vi "Read SCH Parameters MGI RWA.vi"(8 "error in (no error)":errorcluster, 10 "Done":bool, 11 "FPGA Refnum in":T2) -> (0 "error out":errorcluster, 3 "Refnum out":T2)   [LabVIEW 2018]
doc: "Author: Scott Hannahs <sth@magnet.fsu.edu>\nCopyright 2018 Florida State University, All rights reserved."
uses:
  RT Controls/FPGA SCH Digitizer Ref.ctl
  SCH Data Controls/FPGA Configure Parameters.ctl
  <userlib>/_MGI/Read Write Anything/MGI RWA Options Cluster.ctl
panel:
  in  "FPGA Configuration Values":T1={"Ln2 Filter Size"=10, "VT Quench Tick Limit"=4000000, "VT Quench Volt Limit"=0.1000061035156, "Joint Tick Limit"=4000000, "Joint Volt Limit"=0.003, "CoWound Volt Limit"=0.2000122070312, "CoWound Tick Limit"=4000000, "SC Bus Limit"=0.0004000067710876, "SC Bus Tick Limit"=4000000, "ResMag Tick Limit"=1000000, "DAQ Cycle Ticks"=4096, "Res Mag dI/dt Delay"=256, "dI/dT scaling"=38.14697265625, "Pressure Inlet Limit (BarA)"=6.0, "Bore Tube Volt Limit"=0.5999999940395, "Pressure Outlet Limit (BarA)"=5.0, "Activation Current (kA)"=0.5, "Dump Resistor Scale Factor"=250.0625, "Co-Wound Asymmetry Factor"=-0.0026654, "Co-Wound Scale Factor"=60.04379999638, "Layer Scale Factors"=[4.000479996204, 3.501155003905, 3.50127799809, 3.501155003905, 3.001561000943, 3.001561000943, 3.50005300343, 3.500664994121, 3.501155003905, 4.000159993768, 3.999679997563, 4.000159993768, 3.998879998922, 3.999520003796, 3.999679997563, 4.000320002437, 4.00096000731, 4.000640004873], "Fudge Factors"=[0.0486624, 0.0491151, -0.0418637, -0.0149169, 0.0726134, -0.0451977, -0.0032112, -0.0234927, -0.002501, 0.0285479, -0.0270486, 0.003522, 0.0059306, -0.0088003, -0.0297659, 0.0390219], "Joint Scale Factors"=[0.0002005249261856, 0.0002005249261856, 0.0002004057168961, 0.000200480222702, 0.0002004057168961, 0.0002007633447647, 0.0002006888389587, 0.0002006441354752], "SC Bus Scale"=[0.100018, 0.100015, 0.00099996, 0.00099996, 0.0002005249261856, 0.0002006441354752], "Pressure Scale Factor"=[1.723690003157, 1.723690003157, 1.723690003157, 1.723690003157], "# Consecutive Zeros Fault"=1000, "Digitize Convert Ticks"=200, "Digitize Reset Ticks"=400, "Convert Clock Ticks"=20, "Digitize Read Delay Ticks"=38, "Digitize # Bits"=16, "HTS Lead Tick Limit"=4000000, "Res Lead Tick Limit"=4000000, "HTS Lead Trip"=0.1500000059605, "Res Lead Limit"=0.001953125, "HTS Lead FRZ"=0.006999999284744, "HTS Lead Warn"=0.001000002026558, "Low Current (kA)"=0.04500000178814, "Low Current Ticks"=400000000, "Low Current Delay Factor"=100, "HTS Resistance (nOhm)"=[118.0, 131.0], "Ticks to Close Relief"=80000000, "All Breaker Tick Limit"=400000000, "HTS Offset (microV)"=[0.0, 0.0], "Delay Ticks Between Bkr Reset"=1200000000, "Breaker Reset Ticks"=400000000, "PS Enable Reset Ticks"=400000000, "Reset Digitizer Ticks"=400000000, "Pressure Inlet Cooldown Limit"=12.0, "Pressure Outlet Cooldown Limit"=10.0, "Notification Email"="sth@magnet.fsu.edu"} {"Pressure Outlet Cooldown Limit" format="%.5g"; "Pressure Inlet Cooldown Limit" format="%.5g"; "HTS Offset (microV)" format="%_6g"; "HTS Resistance (nOhm)" format="%_6g"; "HTS Lead Warn" format="%_6g"; "HTS Lead FRZ" format="%_6g"; "Res Lead Limit" format="%_6g"; "HTS Lead Trip" format="%_6g"; "Pressure Scale Factor" format="%_6g"; "Joint Scale Factors" format="%_6g"; "Fudge Factors" format="%.7g"; "Co-Wound Asymmetry Factor" format="%.8g"; "Activation Current (kA)" format="%_6g"; "Pressure Outlet Limit (BarA)" format="%.5g"; "Bore Tube Volt Limit" format="%_6g"; "Pressure Inlet Limit (BarA)" format="%.5g"; "dI/dT scaling" format="%.11g"; "SC Bus Limit" format="%_6g"; "Joint Volt Limit" format="%_6g"; "VT Quench Volt Limit" format="%.5g"}
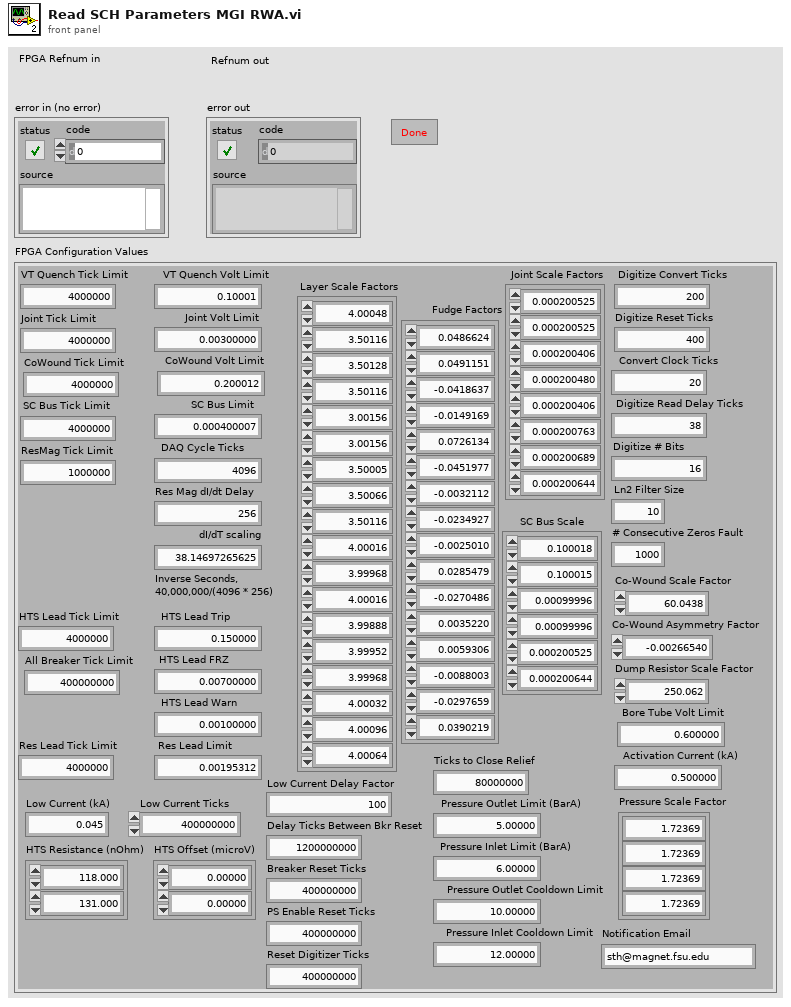
[diagram p1: front panel]
types:
  T1 = typedef "FPGA Configure Parameters.ctl" = cluster{"Ln2 Filter Size":i16, "VT Quench Tick Limit":u32, "VT Quench Volt Limit":dbl, "Joint Tick Limit":u32, "Joint Volt Limit":dbl, "CoWound Volt Limit":dbl, "CoWound Tick Limit":u32, "SC Bus Limit":dbl, "SC Bus Tick Limit":u32, "ResMag Tick Limit":u32, "DAQ Cycle Ticks":u32, "Res Mag dI/dt Delay":u32, "dI/dT scaling":dbl, "Pressure Inlet Limit (BarA)":dbl, "Bore Tube Volt Limit":dbl, "Pressure Outlet Limit (BarA)":dbl, "Activation Current (kA)":dbl, "Dump Resistor Scale Factor":dbl, "Co-Wound Asymmetry Factor":dbl, "Co-Wound Scale Factor":dbl, "Layer Scale Factors":dbl[], "Fudge Factors":dbl[], "Joint Scale Factors":dbl[], "SC Bus Scale":dbl[], "Pressure Scale Factor":dbl[], "# Consecutive Zeros Fault":i16, "Digitize Convert Ticks":u32, "Digitize Reset Ticks":u32, "Convert Clock Ticks":u32, "Digitize Read Delay Ticks":u32, "Digitize # Bits":u32, "HTS Lead Tick Limit":u32, "Res Lead Tick Limit":u32, "HTS Lead Trip":dbl, "Res Lead Limit":dbl, "HTS Lead FRZ":dbl, "HTS Lead Warn":dbl, "Low Current (kA)":dbl, "Low Current Ticks":u32, "Low Current Delay Factor":u16, "HTS Resistance (nOhm)":dbl[], "Ticks to Close Relief":u32, "All Breaker Tick Limit":u32, "HTS Offset (microV)":dbl[], "Delay Ticks Between Bkr Reset":u32, "Breaker Reset Ticks":u32, "PS Enable Reset Ticks":u32, "Reset Digitizer Ticks":u32, "Pressure Inlet Cooldown Limit":dbl, "Pressure Outlet Cooldown Limit":dbl, "Notification Email":string}
  T2 = typedef "FPGA SCH Digitizer Ref.ctl" = refnum<k20>
  T3 = typedef "MGI RWA Options Cluster.ctl" = cluster{"TS Fmt":string, "Int Fmt":string, "Delimiter":string}
  T4 = cluster{"Ln2 Filter Size":i16, "VT Quench Tick Limit":u32, "VT Quench Volt Limit":dbl, "Joint Tick Limit":u32, "Joint Volt Limit":dbl, "CoWound Volt Limit":dbl, "CoWound Tick Limit":u32, "SC Bus Limit":dbl, "SC Bus Tick Limit":u32, "ResMag Tick Limit":u32, "DAQ Cycle Ticks":u32, "Res Mag dI/dt Delay":u32, "dI/dT scaling":dbl, "Pressure Inlet Limit (BarA)":dbl, "Bore Tube Volt Limit":dbl, "Pressure Outlet Limit (BarA)":dbl, "Activation Current (kA)":dbl, "Dump Resistor Scale Factor":dbl, "Co-Wound Asymmetry Factor":dbl, "Co-Wound Scale Factor":dbl, "Layer Scale Factors":dbl[], "Fudge Factors":dbl[], "Joint Scale Factors":dbl[], "SC Bus Scale":dbl[], "Pressure Scale Factor":dbl[], "# Consecutive Zeros Fault":i16, "Digitize Convert Ticks":u32, "Digitize Reset Ticks":u32, "Convert Clock Ticks":u32, "Digitize Read Delay Ticks":u32, "Digitize # Bits":u32, "HTS Lead Tick Limit":u32, "Res Lead Tick Limit":u32, "HTS Lead Trip":dbl, "Res Lead Limit":dbl, "HTS Lead FRZ":dbl, "HTS Lead Warn":dbl, "Low Current (kA)":dbl, "Low Current Ticks":u32, "Low Current Delay Factor":u16, "HTS Resistance (nOhm)":dbl[], "Ticks to Close Relief":u32, "All Breaker Tick Limit":u32, "HTS Offset (microV)":dbl[], "Delay Ticks Between Bkr Reset":u32, "Breaker Reset Ticks":u32, "PS Enable Reset Ticks":u32, "Reset Digitizer Ticks":u32, "Pressure Inlet Cooldown Limit":dbl, "Pressure Outlet Cooldown Limit":dbl, "Notification Email":string}
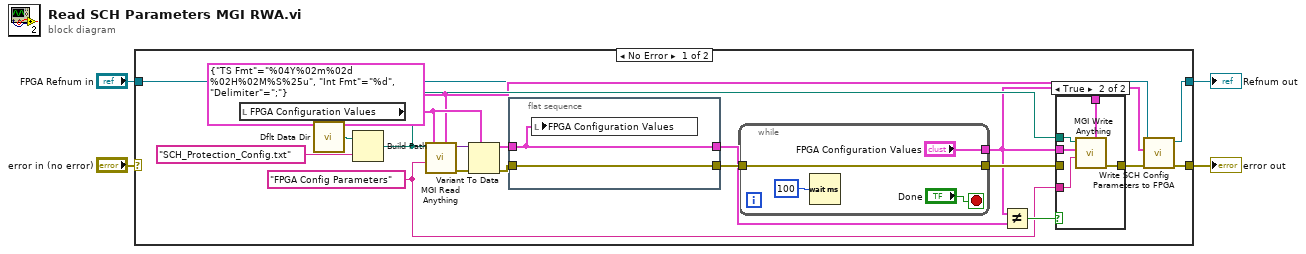
[diagram p0: block diagram]
diagram:
  n1 = case shown="No Error" "error in (no error)" {
    selector: "error in (no error)" -> [_ w37]
    tunnel: [w10 w37] -> w3
    tunnel: "FPGA Refnum in" -> [w5 w36]
    tunnel: [w8 w36] -> w1
    frame No Error {
      w6 = T3 {"TS Fmt"="%04Y%02m%02d %02H%02M%S%25u", "Int Fmt"="%d", "Delimiter"=";"} ("Read/Write Options (Version 1.x)")
      w13 = "FPGA Config Parameters" ("section")
      n2 = local read "FPGA Configuration Values"() -> (w16:T1)
      n3 = call <vilib>:"Dflt Data Dir.vi"() -> ("App:Default Data Directory"=w23:path)
      n4 = Build Path(base path=w23, name or relative path="SCH_Protection_Config.txt") -> (appended path=w12:path)
      n5 = call <userlib>:"MGI Read Anything.vi"("Read/Write Options (Version 1.x)"=w6, "Type of Anything"=w16, "Section Name (Name of \"Type of Anything\")"=w13, "Path (dialog)"=w12) -> ("Error Out"=w7:errorcluster, "Anything"=w17:variant)  [unwired: 4 in, 2 out]
      n6 = Variant To Data(error in=w7, type=w16, Variant=w17) -> (data=w15:T4, error out=w14:errorcluster)
      n7 = flat-sequence {
        tunnel: [w24] -> w21
        tunnel: [w25] -> w20
        tunnel: w15 -> [w25]
        tunnel: w14 -> [w24]
        frame #0 {
          n8 = local write "FPGA Configuration Values"(w25) -> ()
        }
      }
      n9 = while {
        tunnel: w21 -> [w35]
        tunnel: [w35] -> w18
        tunnel: ["FPGA Configuration Values"] -> w9
        stop <- "Done" stop-if-true
        n10 = Wait (ms)(milliseconds to wait=u32 100) -> ()  [unwired: 1 out]
      }
      n11 = Not Equal?(x=w9, y=w20) -> (x != y?=w19:bool)
      n12 = case shown="True" w19 {
        tunnel: w18 -> [w26 _]
        tunnel: w9 -> [_ w28]
        tunnel: [w26 w29] -> w11
        tunnel: w13 -> [_ w31]
        tunnel: w12 -> [_ w30]
        tunnel: w6 -> [_ w27]
        frame False {
        }
        frame True {
          n13 = call <userlib>:"MGI Write Anything.vi"("Read/Write Options"=w27, "Section Name (Name of \"Anything\")"=w31, "Anything"=w28, "Path (dialog)"=w30) -> ("Error Out"=w29:errorcluster)  [unwired: 5 in, 2 out]
        }
      }
      n14 = call "Write SCH Config Parameters to FPGA.vi"("error in (no error)"=w11, "FPGA Configuration Values"=w9, "Refnum in"=w5) -> ("error out"=w10:errorcluster, "Refnum out"=w8:T2)  [unwired: 7 in]
    }
    frame Error {
    }
  }
  "Refnum out" <- w1
  "error out" <- w3
